vi "Query Active DUT Airplane Mode Actions State.vi"(8 "error in (no error)":errorcluster, 11 "VISA resource name":refnum<visa-resource-name>) -> (0 "error out":errorcluster, 1 "Switch Off":i32, 2 "Switch On":i32, 3 "VISA resource name out":refnum<visa-resource-name>)   [LabVIEW 2020, in "Rohde&Schwarz CMXP Base.lvlib"]
doc: "Queries the states of airplane mode actions.\n\nAttribute:\n-\n\nRemote-control command:\nFETCh:DUT:CONTrol:AIRPlane:STATe?"
uses:
  <instrlib>/Rohde&Schwarz CMXP Base/Rohde&Schwarz CMXP Base.lvlib
  <instrlib>/Rohde&Schwarz CMXP Base/Private/rsidr_core.llb/rsidr_core.lvlib
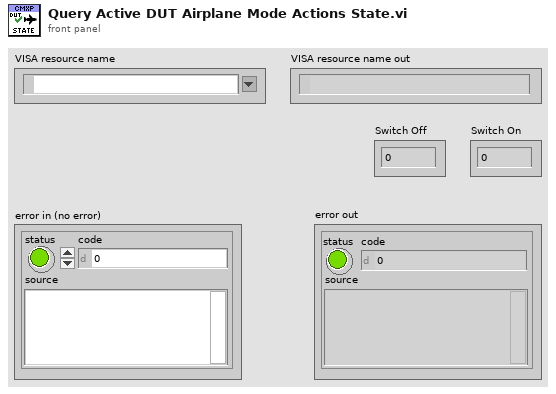
[diagram p1: front panel]
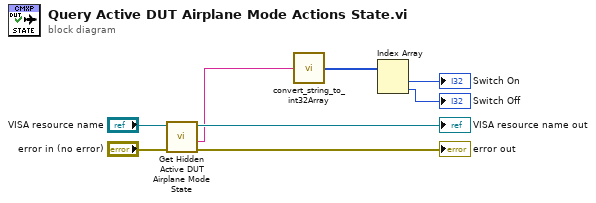
[diagram p0: block diagram]
diagram:
  n1 = call "Get Hidden Active DUT Airplane Mode State"("error in (no error)"="error in (no error)", "instrument handle"="VISA resource name") -> ("error out"=→"error out":errorcluster, "Hidden Active DUT Airplane Mode State"=w1:string, "instrument handle out"=→"VISA resource name out":refnum<visa-resource-name>)  [unwired: 7 in]
  n2 = call <instrlib>:"convert_string_to_int32Array.vi"("string in"=w1) -> ("int32 array out"=w4:i32[])  [unwired: 3 in, 1 out]
  n3 = Index Array(array=w4) -> (element #1=→"Switch On":i32, element #2=→"Switch Off":i32)  [unwired: 2 in]
